vi "LPA400_check_strip_cheksum.vi"(0 "LPA400 individual scale string":string="#X01+234J@!") -> (1 "Cleaned good string":string, 2 "Error Notes":string)   [LabVIEW 2010]
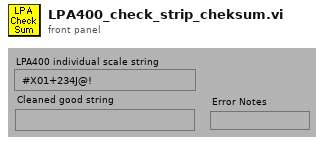
[diagram p1: front panel]
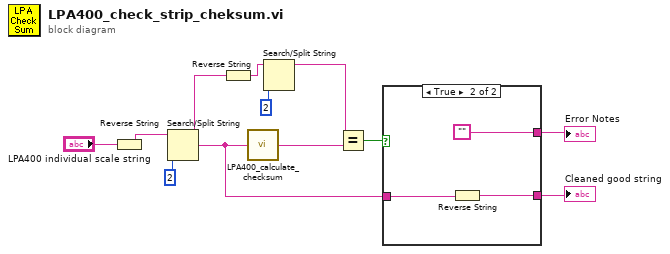
[diagram p0: block diagram]
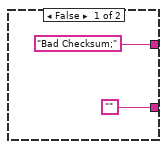
[diagram p2: hidden frame]
diagram:
  n1 = Reverse String(1:"LPA400 individual scale string") -> (0:w11:string)
  n2 = Search/Split String(string=w11, offset (0)=2) -> (substring before match=w9:string, match + rest of string=w3:string)  [unwired: 2 out]
  n3 = Reverse String(1:w9) -> (0:w7:string)
  n4 = call "LPA400_calculate_checksum.vi"("String"=w3) -> ("Checksum"=w5:string)
  n5 = Search/Split String(string=w7, offset (0)=2) -> (substring before match=w6:string)  [unwired: 3 out]
  n6 = Equal?(x=w6, y=w5) -> (x = y?=w4:bool)
  n7 = case shown="True" w4 {
    tunnel: w3 -> [_ w17]
    tunnel: ["" w16] -> w2
    tunnel: ["Bad Checksum;" ("f") ""] -> w1
    frame False {
    }
    frame True {
      n8 = Reverse String(1:w17) -> (0:w16:string)
    }
  }
  "Error Notes" <- w1
  "Cleaned good string" <- w2
